vi "IIC Write Read Bytes Of Event.vi"(0 "DevIndex":i32, 1 "WriteLen":i32, 2 "EventPin":i32, 3 "TimeOutOfEventMs":i32, 5 "IICIndex":i32, 7 "SlaveAddr":i16, 9 "pWriteData":u8[](array[numeric])=array[20480 elements], 12 "ReadLen":i32, 13 "EventType":u8) -> (4 "pReadData":u8[](array[numeric]), 6 "function return":i32)   [LabVIEW 2010, in "usb2iic.lvlib"]
doc: "int WINAPI IIC_WriteReadBytesOfEvent(int DevIndex,int IICIndex,short SlaveAddr,unsigned char *pWriteData,int WriteLen,unsigned char *pReadData,int ReadLen,int EventPin,unsigned char EventType,int TimeOutOfEventMs);"
uses:
  usb2iic.lvlib
  USB2XXX.dll
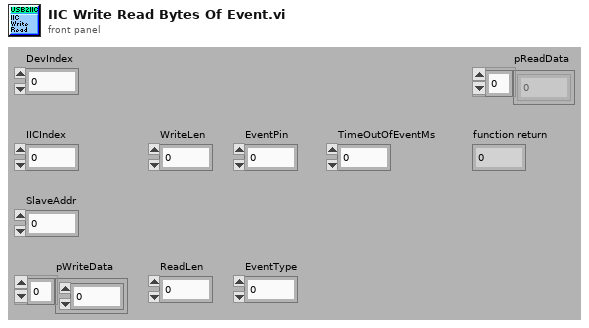
[diagram p1: front panel]
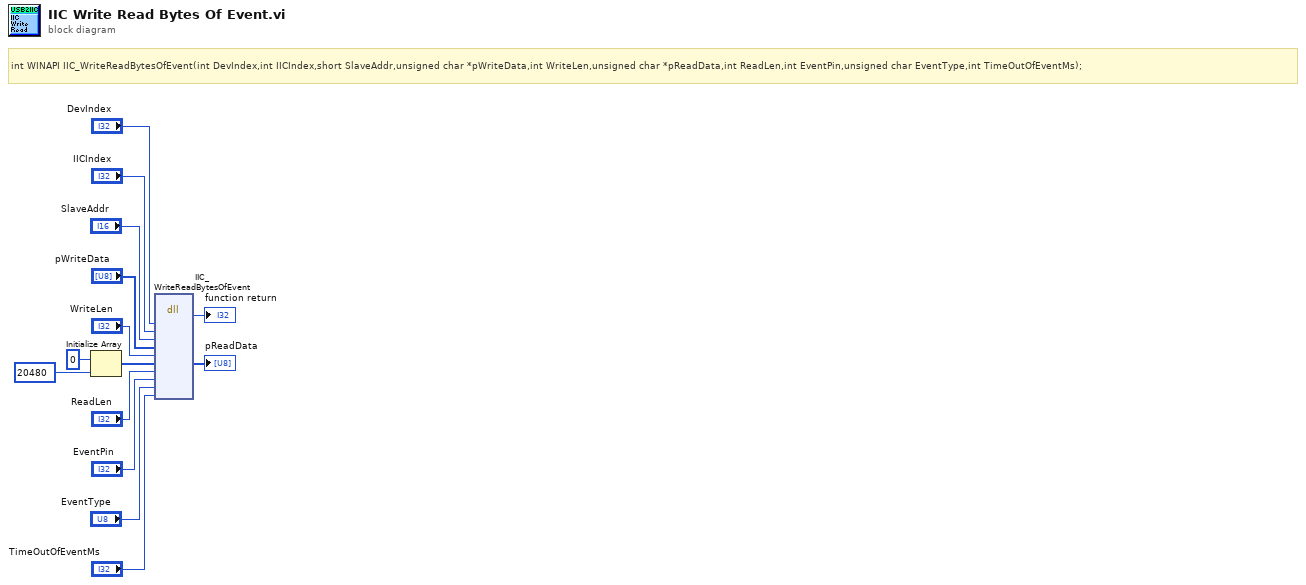
[diagram p0: block diagram]
diagram:
  # "int WINAPI IIC_WriteReadBytesOfEvent(int DevIndex,int IICIndex,short SlaveAddr,unsigned char *pWriteData,int WriteLen,unsigned char *pReadData,int ReadLen,int EventPin,unsigned char EventType,int TimeOutOfEventMs);"
  n1 = Initialize Array(u8 0 ("element"), 20480 ("dimension size")) -> (w8:u8[])
  n2 = dll-call lib="G:/OtherWork/USB2XXX_Example/trunk/Labview/PublicFiles/usb2iic/USB2XXX.*" fn="IIC_WriteReadBytesOfEvent"("DevIndex"="DevIndex", "IICIndex"="IICIndex", "SlaveAddr"="SlaveAddr", "pWriteData"="pWriteData", "WriteLen"="WriteLen", "pReadData"=w8, "ReadLen"="ReadLen", "EventPin"="EventPin", "EventType"="EventType", "TimeOutOfEventMs"="TimeOutOfEventMs") -> (→"function return":i32, "pReadData"=→"pReadData":u8[])  [unwired: 12 in, 2 out]
